vi "CheckSettings.vi"(8 "error in (no error)":errorcluster, 11 "NHRDCPower in":refnum<class "NHRDCPower.lvclass">) -> (0 "error out":errorcluster, 3 "NHRDCPower out":refnum<class "NHRDCPower.lvclass">)   [LabVIEW 2018, in "AcPwrPlugins.lvlib" / "NHRDCPower.lvclass"]
uses:
  NHRDCPower.lvclass
  C:/Users/ico/Documents/Projects/NistPluggableModules/AcPwr/AcPwrPlugins/AcPwrBaseClass/AcPwrBase.lvclass
  TypeDefs/CheckSettings.ctl
  <vilib>/Utility/error.llb/Error Cluster From Error Code.vi
  <vilib>/ErrorRing/Error Ring.xnode
  <instrlib>/NHRDCPowerModule/NHRDCPowerModule/NHRDCPowerModule.lvlib
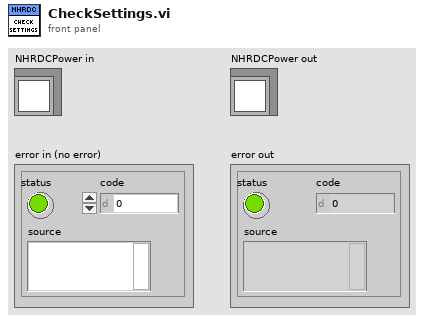
[diagram p1: front panel]
types:
  T1 = typedef "AcPwrPlugins.lvlib/NHRDCPower.lvclass/CheckSettings.ctl" = enum16{"Aperture", "Voltage", "Voltage Slew Rate", "Current", "Current Slew Rate", "Resistance", "Resistance Slew Rate", "Power", "Power Slew Rate", "RefreshTime"}
  T2 = typedef "AcPwrPlugins.lvlib/NHRDCPower.lvclass/Device(s)Settings.ctl" = cluster{"Handle":string, "Name":string, "id query (Yes)":bool, "reset device (Yes)":bool, "Connected":bool, "Voltage Range (V)":dbl[], "Timing":cluster{"TimingOn":enum16{""}, "Hours":u32, "Minutes":u32, "Seconds":dbl, "CutoffVoltage":dbl}, "Initial Battery Detect Voltage (0)":dbl, "SafetySettings":cluster{"SetWatchDog":bool, "Voltage (V)":sgl, "Current (A)":sgl, "Power (W)":sgl, "Voltage Delay (s)":sgl, "Current Delay (s)":sgl, "Power Delay (s)":sgl}, "Options String":string, "Aperture Time (s)":sgl, "operating state (Off)":i32, "OutputSettings":cluster{"Voltage (V)":sgl, "Current (A)":sgl, "Resistance (Ohms)":sgl, "Power (W)":sgl, "Enable Voltage":bool, "Enable Current":bool, "Enable Resistance":bool, "Enable Power":bool, "Delay After (s)":sgl}[], "SlewRate":cluster{"Set Voltage Rate V/S":sgl, "Set Current Rate A/S":sgl, "Set Resistance Rate R/S":sgl, "Set Power Rate W/S":sgl}}[]
  T3 = cluster{"Set Voltage Rate V/S":sgl, "Set Current Rate A/S":sgl, "Set Resistance Rate R/S":sgl, "Set Power Rate W/S":sgl}
  T4 = cluster{"Voltage (V)":sgl, "Current (A)":sgl, "Resistance (Ohms)":sgl, "Power (W)":sgl, "Enable Voltage":bool, "Enable Current":bool, "Enable Resistance":bool, "Enable Power":bool, "Delay After (s)":sgl}[]
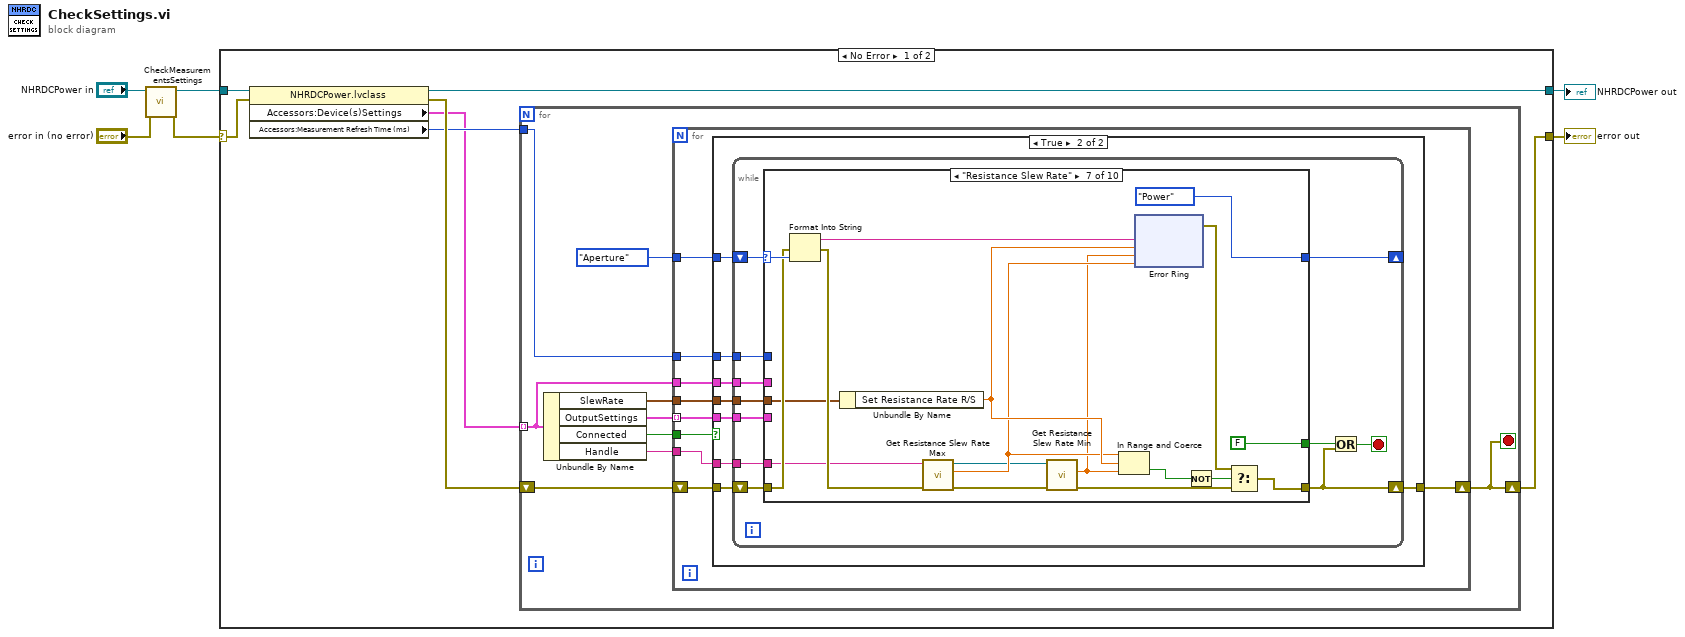
[diagram p0: block diagram]
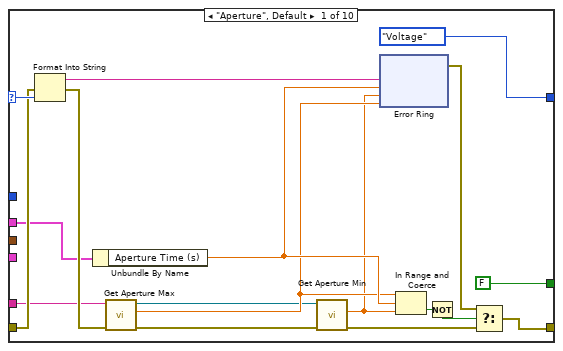
[diagram p3: hidden frame]
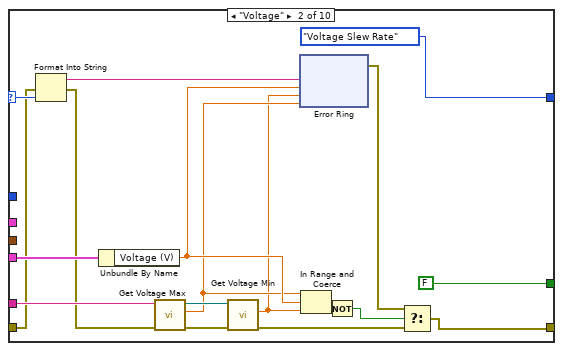
[diagram p4: hidden frame]
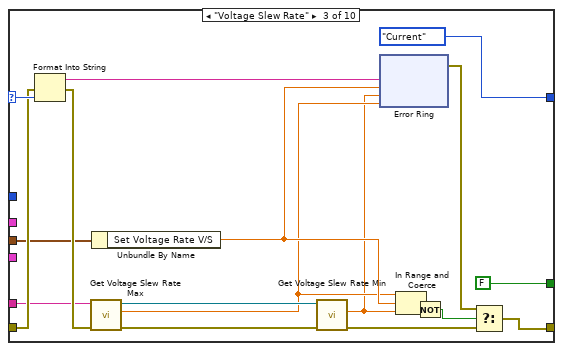
[diagram p5: hidden frame]
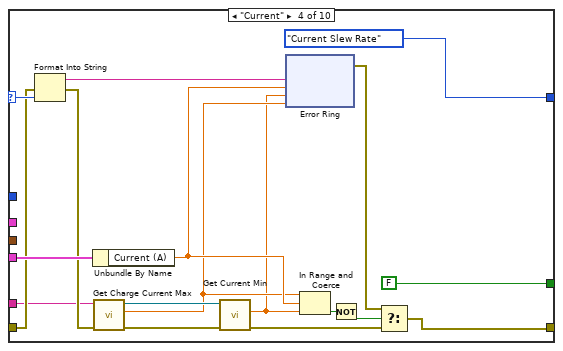
[diagram p6: hidden frame]
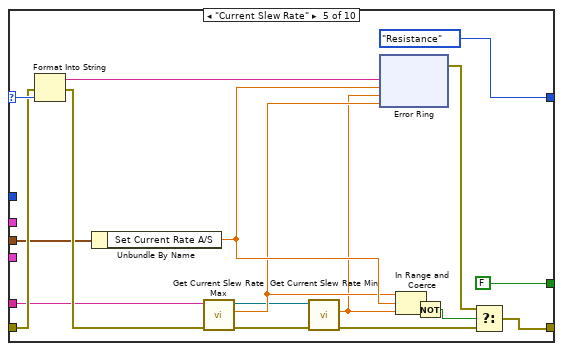
[diagram p7: hidden frame]
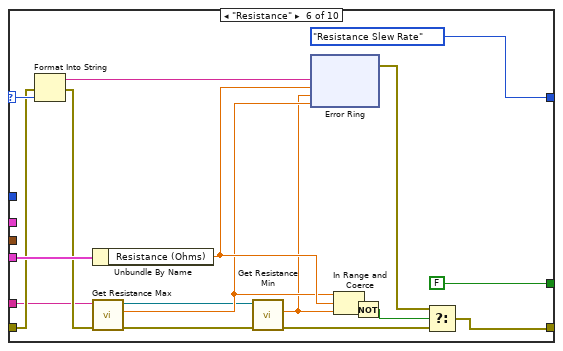
[diagram p8: hidden frame]
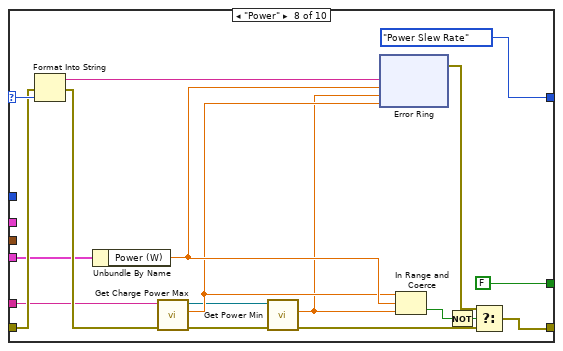
[diagram p9: hidden frame]
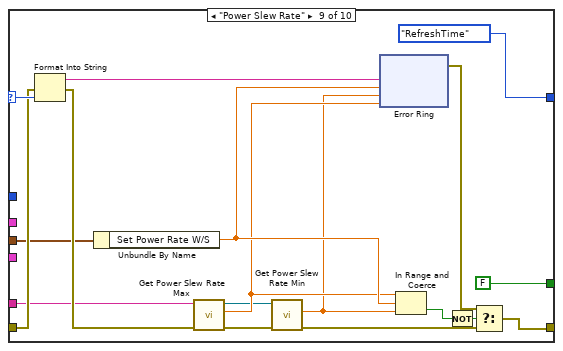
[diagram p10: hidden frame]
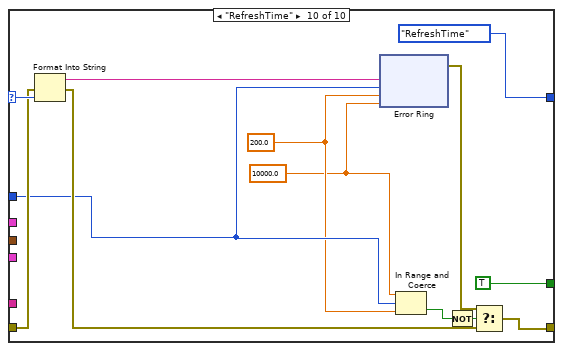
[diagram p11: hidden frame]
diagram:
  n1 = call-dynamic "CheckMeasurementsSettings.vi"("error in (no error)"="error in (no error)", "NHRDCPower in"="NHRDCPower in") -> ("error out"=w1:errorcluster, "NHRDCPower out"=w2:refnum<class "NHRDCPower.lvclass">)  [unwired: 8 in]
  n2 = case shown="No Error" w1 {
    selector: w1 -> [w12 w328]
    tunnel: [w11 w328] -> w5
    tunnel: [w13 w327] -> w6
    tunnel: w2 -> [w9 w327]
    frame No Error {
      n3 = property class="NHRDCPower.lvclass"(reference=w9, error in=w12) -> (reference out=w13:refnum<class "NHRDCPower.lvclass">, error out=w10:errorcluster, "Accessors:Device(s)Settings"=w7:T2, "Accessors:Measurement Refresh Time (ms)"=w8:u32)
      n4 = for {
        tunnel: w7 -> [w14] mode=indexing
        shift-right: [w22] -> w11
        shift-left: w10 -> [w17]
        tunnel: w8 -> [w15]
        stop <- w22 stop-if-true
        n5 = Unbundle By Name(w14) -> ("SlewRate"=w18:T3, "OutputSettings"=w19:T4, "Connected"=w20:bool, "Handle"=w21:string)
        n6 = for {
          tunnel: w21 -> [w30]
          tunnel: w20 -> [w29]
          tunnel: w19 -> [w28] mode=indexing
          tunnel: w18 -> [w27]
          tunnel: CheckSettings."Aperture" ("CheckSettings Enum") -> [w25]
          tunnel: w15 -> [w24]
          shift-right: [w31] -> w22
          shift-left: w17 -> [w26]
          tunnel: w14 -> [w23]
          n7 = case shown="True" w29 {
            tunnel: w26 -> [w32 w40]
            tunnel: [w32 w37] -> w31
            tunnel: w30 -> [_ w39]
            tunnel: w28 -> [_ w38]
            tunnel: w27 -> [_ w35]
            tunnel: w25 -> [_ w36]
            tunnel: w24 -> [_ w34]
            tunnel: w23 -> [_ w33]
            frame False {
            }
            frame True {
              n8 = while {
                tunnel: w39 -> [w50]
                tunnel: w38 -> [w49]
                shift-right: [w45] -> w37
                shift-left: w40 -> [w51]
                shift-right: [w44] -> _
                shift-left: w36 -> [w48]
                tunnel: w35 -> [w43]
                tunnel: w34 -> [w42]
                tunnel: w33 -> [w41]
                stop <- w47 stop-if-true
                n9 = case shown="\"Resistance Slew Rate\"" w48 {
                  selector: w48 -> [w64 w85 w120 w147 w176 w203 w232 w260 w289 w312]
                  tunnel: w51 -> [w63 w84 w119 w146 w175 w202 w231 w259 w288 w311]
                  tunnel: w50 -> [w59 w97 w116 w141 w172 w199 w228 w256 w285 _]
                  tunnel: w49 -> [_ w94 _ w153 _ w209 _ w254 _ _]
                  tunnel: [w68 w89 w124 w151 w180 w207 w236 w264 w293 w316] -> w45
                  tunnel: [FALSE FALSE FALSE FALSE FALSE FALSE FALSE FALSE FALSE TRUE] -> w46
                  tunnel: [CheckSettings."Voltage" ("CheckSettings Enum") CheckSettings."Voltage Slew Rate" ("CheckSettings Enum") CheckSettings."Current" ("CheckSettings Enum") CheckSettings."Current Slew Rate" ("CheckSettings Enum") CheckSettings."Resistance" ("CheckSettings Enum") CheckSettings."Resistance Slew Rate" ("CheckSettings Enum") CheckSettings."Power" ("CheckSettings Enum") CheckSettings."Power Slew Rate" ("CheckSettings Enum") CheckSettings."RefreshTime" ("CheckSettings Enum") CheckSettings."RefreshTime" ("CheckSettings Enum")] -> w44
                  tunnel: w43 -> [_ _ w109 _ w170 _ w226 _ w283 _]
                  tunnel: w42 -> [_ _ _ _ _ _ _ _ _ w306]
                  tunnel: w41 -> [w52 _ _ _ _ _ _ _ _ _]
                  frame "Aperture", Default {
                    n10 = Format Into String(error in=w63, w64) -> (resulting string=w61:string, error out=w62:errorcluster)  [unwired: 2 in]
                    n11 = Unbundle By Name(w52) -> ("Aperture Time (s)"=w69:sgl)
                    n12 = call <instrlib>:"Get Aperture Max.vi"("error in (no error)"=w62, "instrument handle"=w59) -> ("error out"=w60:errorcluster, "maximum aperture"=w58:sgl, "instrument handle out"=w57:refnum<visa-resource-name>)  [unwired: 7 in]
                    n13 = call <instrlib>:"Get Aperture Min.vi"("error in (no error)"=w60, "instrument handle"=w57) -> ("error out"=w55:errorcluster, "minimum aperture"=w56:sgl)  [unwired: 7 in, 1 out]
                    n14 = xnode "Error Ring"("parameter 0"=w61, "parameter 1"=w69, "parameter 2"=w56, "parameter 3"=w58) -> ("error out"=w67:errorcluster)
                    n15 = In Range and Coerce(upper limit=w58, x=w69, lower limit=w56) -> (In Range?=w66:bool)  [unwired: 1 out]
                    n16 = Not(x=w66) -> (.not. x?=w53:bool)
                    n17 = Select(t=w67, s=w53, f=w55) -> (s? t:f=w68:errorcluster)
                  }
                  frame "Voltage" {
                    n18 = Format Into String(error in=w84, w85) -> (resulting string=w82:string, error out=w83:errorcluster)  [unwired: 2 in]
                    n19 = Unbundle By Name(w94) -> ("Voltage (V)"=w93:sgl)
                    n20 = call <instrlib>:"Get Voltage Max.vi"("error in (no error)"=w83, "instrument handle"=w97) -> ("error out"=w95:errorcluster, "maximum voltage"=w92:sgl, "instrument handle out"=w96:refnum<visa-resource-name>)  [unwired: 7 in]
                    n21 = call <instrlib>:"Get Voltage Min.vi"("error in (no error)"=w95, "instrument handle"=w96) -> ("error out"=w90:errorcluster, "minimum voltage"=w91:sgl)  [unwired: 7 in, 1 out]
                    n22 = xnode "Error Ring"("parameter 0"=w82, "parameter 1"=w93, "parameter 2"=w91, "parameter 3"=w92) -> ("error out"=w88:errorcluster)
                    n23 = In Range and Coerce(upper limit=w92, x=w93, lower limit=w91) -> (In Range?=w87:bool)  [unwired: 1 out]
                    n24 = Not(x=w87) -> (.not. x?=w80:bool)
                    n25 = Select(t=w88, s=w80, f=w90) -> (s? t:f=w89:errorcluster)
                  }
                  frame "Voltage Slew Rate" {
                    n26 = Format Into String(error in=w119, w120) -> (resulting string=w117:string, error out=w118:errorcluster)  [unwired: 2 in]
                    n27 = call <instrlib>:"Get Voltage Slew Rate Max.vi"("error in (no error)"=w118, "instrument handle"=w116) -> ("error out"=w114:errorcluster, "maximum voltage slew rate"=w111:sgl, "instrument handle out"=w112:refnum<visa-resource-name>)  [unwired: 7 in]
                    n28 = Unbundle By Name(w109) -> ("Set Voltage Rate V/S"=w125:sgl)
                    n29 = call <instrlib>:"Get Voltage Slew Rate Min.vi"("error in (no error)"=w114, "instrument handle"=w112) -> ("error out"=w113:errorcluster, "minimum voltage slew rate"=w110:sgl)  [unwired: 7 in, 1 out]
                    n30 = xnode "Error Ring"("parameter 0"=w117, "parameter 1"=w125, "parameter 2"=w110, "parameter 3"=w111) -> ("error out"=w123:errorcluster)
                    n31 = In Range and Coerce(upper limit=w111, x=w125, lower limit=w110) -> (In Range?=w122:bool)  [unwired: 1 out]
                    n32 = Not(x=w122) -> (.not. x?=w108:bool)
                    n33 = Select(t=w123, s=w108, f=w113) -> (s? t:f=w124:errorcluster)
                  }
                  frame "Current" {
                    n34 = Format Into String(error in=w146, w147) -> (resulting string=w144:string, error out=w145:errorcluster)  [unwired: 2 in]
                    n35 = Unbundle By Name(w153) -> ("Current (A)"=w152:sgl)
                    n36 = call <instrlib>:"Get Charge Current Max.vi"("error in (no error)"=w145, "instrument handle"=w141) -> ("error out"=w142:errorcluster, "charge current max"=w139:sgl, "instrument handle out"=w140:refnum<visa-resource-name>)  [unwired: 7 in]
                    n37 = call <instrlib>:"Get Current Min.vi"("error in (no error)"=w142, "instrument handle"=w140) -> ("error out"=w143:errorcluster, "minimum current"=w138:sgl)  [unwired: 7 in, 1 out]
                    n38 = xnode "Error Ring"("parameter 0"=w144, "parameter 1"=w152, "parameter 2"=w138, "parameter 3"=w139) -> ("error out"=w150:errorcluster)
                    n39 = In Range and Coerce(upper limit=w139, x=w152, lower limit=w138) -> (In Range?=w149:bool)  [unwired: 1 out]
                    n40 = Not(x=w149) -> (.not. x?=w136:bool)
                    n41 = Select(t=w150, s=w136, f=w143) -> (s? t:f=w151:errorcluster)
                  }
                  frame "Current Slew Rate" {
                    n42 = Format Into String(error in=w175, w176) -> (resulting string=w173:string, error out=w174:errorcluster)  [unwired: 2 in]
                    n43 = Unbundle By Name(w170) -> ("Set Current Rate A/S"=w181:sgl)
                    n44 = call <instrlib>:"Get Current Slew Rate Max.vi"("error in (no error)"=w174, "instrument handle"=w172) -> ("error out"=w169:errorcluster, "maximum current slew rate"=w168:sgl, "instrument handle out"=w166:refnum<visa-resource-name>)  [unwired: 7 in]
                    n45 = call <instrlib>:"Get Current Slew Rate Min.vi"("error in (no error)"=w169, "instrument handle"=w166) -> ("error out"=w167:errorcluster, "minimum current slew rate"=w165:sgl)  [unwired: 7 in, 1 out]
                    n46 = xnode "Error Ring"("parameter 0"=w173, "parameter 1"=w181, "parameter 2"=w165, "parameter 3"=w168) -> ("error out"=w179:errorcluster)
                    n47 = In Range and Coerce(upper limit=w168, x=w181, lower limit=w165) -> (In Range?=w178:bool)  [unwired: 1 out]
                    n48 = Not(x=w178) -> (.not. x?=w164:bool)
                    n49 = Select(t=w179, s=w164, f=w167) -> (s? t:f=w180:errorcluster)
                  }
                  frame "Resistance" {
                    n50 = Format Into String(error in=w202, w203) -> (resulting string=w200:string, error out=w201:errorcluster)  [unwired: 2 in]
                    n51 = Unbundle By Name(w209) -> ("Resistance (Ohms)"=w208:sgl)
                    n52 = call <instrlib>:"Get Resistance Max.vi"("error in (no error)"=w201, "instrument handle"=w199) -> ("error out"=w198:errorcluster, "maximum resistance"=w197:sgl, "instrument handle out"=w195:refnum<visa-resource-name>)  [unwired: 7 in]
                    n53 = call <instrlib>:"Get Resistance Min.vi"("error in (no error)"=w198, "instrument handle"=w195) -> ("error out"=w196:errorcluster, "minimum resistance"=w194:sgl)  [unwired: 7 in, 1 out]
                    n54 = xnode "Error Ring"("parameter 0"=w200, "parameter 1"=w208, "parameter 2"=w194, "parameter 3"=w197) -> ("error out"=w206:errorcluster)
                    n55 = In Range and Coerce(upper limit=w197, x=w208, lower limit=w194) -> (In Range?=w205:bool)  [unwired: 1 out]
                    n56 = Not(x=w205) -> (.not. x?=w192:bool)
                    n57 = Select(t=w206, s=w192, f=w196) -> (s? t:f=w207:errorcluster)
                  }
                  frame "Resistance Slew Rate" {
                    n58 = Format Into String(error in=w231, w232) -> (resulting string=w229:string, error out=w230:errorcluster)  [unwired: 2 in]
                    n59 = Unbundle By Name(w226) -> ("Set Resistance Rate R/S"=w237:sgl)
                    n60 = call <instrlib>:"Get Resistance Slew Rate Max.vi"("error in (no error)"=w230, "instrument handle"=w228) -> ("error out"=w225:errorcluster, "maximum resistance slew rate"=w224:sgl, "instrument handle out"=w221:refnum<visa-resource-name>)  [unwired: 7 in]
                    n61 = call <instrlib>:"Get Resistance Slew Rate Min.vi"("error in (no error)"=w225, "instrument handle"=w221) -> ("error out"=w223:errorcluster, "minimum resistance slew rate"=w222:sgl)  [unwired: 7 in, 1 out]
                    n62 = In Range and Coerce(upper limit=w224, x=w237, lower limit=w222) -> (In Range?=w234:bool)  [unwired: 1 out]
                    n63 = xnode "Error Ring"("parameter 0"=w229, "parameter 1"=w237, "parameter 2"=w222, "parameter 3"=w224) -> ("error out"=w235:errorcluster)
                    n64 = Not(x=w234) -> (.not. x?=w220:bool)
                    n65 = Select(t=w235, s=w220, f=w223) -> (s? t:f=w236:errorcluster)
                  }
                  frame "Power" {
                    n66 = Format Into String(error in=w259, w260) -> (resulting string=w257:string, error out=w258:errorcluster)  [unwired: 2 in]
                    n67 = Unbundle By Name(w254) -> ("Power (W)"=w265:sgl)
                    n68 = call <instrlib>:"Get Charge Power Max.vi"("error in (no error)"=w258, "instrument handle"=w256) -> ("error out"=w253:errorcluster, "charge power max"=w252:sgl, "instrument handle out"=w249:refnum<visa-resource-name>)  [unwired: 7 in]
                    n69 = call <instrlib>:"Get Power Min.vi"("error in (no error)"=w253, "instrument handle"=w249) -> ("error out"=w251:errorcluster, "minimum power"=w250:sgl)  [unwired: 7 in, 1 out]
                    n70 = xnode "Error Ring"("parameter 0"=w257, "parameter 1"=w265, "parameter 2"=w250, "parameter 3"=w252) -> ("error out"=w263:errorcluster)
                    n71 = In Range and Coerce(upper limit=w252, x=w265, lower limit=w250) -> (In Range?=w262:bool)  [unwired: 1 out]
                    n72 = Not(x=w262) -> (.not. x?=w248:bool)
                    n73 = Select(t=w263, s=w248, f=w251) -> (s? t:f=w264:errorcluster)
                  }
                  frame "Power Slew Rate" {
                    n74 = Format Into String(error in=w288, w289) -> (resulting string=w286:string, error out=w287:errorcluster)  [unwired: 2 in]
                    n75 = Unbundle By Name(w283) -> ("Set Power Rate W/S"=w282:sgl)
                    n76 = call <instrlib>:"Get Power Slew Rate Max.vi"("error in (no error)"=w287, "instrument handle"=w285) -> ("error out"=w281:errorcluster, "maximum power slew rate"=w280:sgl, "instrument handle out"=w278:refnum<visa-resource-name>)  [unwired: 7 in]
                    n77 = call <instrlib>:"Get Power Slew Rate Min.vi"("error in (no error)"=w281, "instrument handle"=w278) -> ("error out"=w279:errorcluster, "minimum power slew rate"=w277:sgl)  [unwired: 7 in, 1 out]
                    n78 = xnode "Error Ring"("parameter 0"=w286, "parameter 1"=w282, "parameter 2"=w277, "parameter 3"=w280) -> ("error out"=w292:errorcluster)
                    n79 = In Range and Coerce(upper limit=w280, x=w282, lower limit=w277) -> (In Range?=w291:bool)  [unwired: 1 out]
                    n80 = Not(x=w291) -> (.not. x?=w276:bool)
                    n81 = Select(t=w292, s=w276, f=w279) -> (s? t:f=w293:errorcluster)
                  }
                  frame "RefreshTime" {
                    w304 = 10000.0 ("parameter 2")
                    w305 = 200.0 ("parameter 2")
                    n82 = Format Into String(error in=w311, w312) -> (resulting string=w309:string, error out=w310:errorcluster)  [unwired: 2 in]
                    n83 = xnode "Error Ring"("parameter 0"=w309, "parameter 1"=w306, "parameter 2"=w305, "parameter 3"=w304) -> ("error out"=w315:errorcluster)
                    n84 = In Range and Coerce(upper limit=w304, x=w306, lower limit=w305) -> (In Range?=w314:bool)  [unwired: 1 out]
                    n85 = Not(x=w314) -> (.not. x?=w307:bool)
                    n86 = Select(t=w315, s=w307, f=w310) -> (s? t:f=w316:errorcluster)
                  }
                }
                n87 = Or(x=w46, y=w45) -> (x .or. y?=w47:bool)
              }
            }
          }
        }
      }
    }
    frame Error {
    }
  }
  "error out" <- w5
  "NHRDCPower out" <- w6
